vi "Get Element Description Variant.vi"(8 "error in (no error)":errorcluster, 9 "Prepend Array Size":bool=TRUE, 11 "Data Type":variant) -> (0 "error out (no error)":errorcluster, 2 "Total Size":u32, 3 "Encoder Data":T1)   [LabVIEW 2021, in "CIF_NI_CIPC.lvlib"]
uses:
  CIF_NI_CIPC.lvlib
  TypeDefs/Encoder Info.ctl
  TypeDefs/Errors.ctl
  <vilib>/CIF Foundation/CIF Utilities/Errors/Append Error Location.vi
  <vilib>/CIF Foundation/CIF Utilities/DataTypes/DataTypes_CIF_U.lvlib
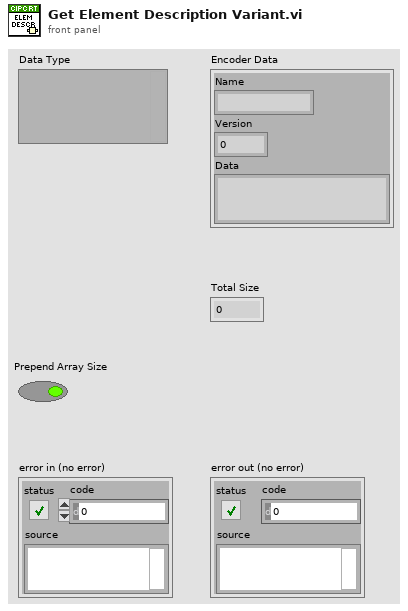
[diagram p1: front panel]
types:
  T1 = typedef "CIF_NI_CIPC.lvlib/Encoder Info.ctl" = cluster{"Name":string, "Version":i32, "Data":string}
  T2 = typedef "DataTypes_CIF_U.lvlib/Cluster Info.ctl" = cluster{"Name":string[], "Indices":i32[], "Type":T3, "Flat Data Size":u32, "Flat Data Offset":u32, "Memory Size":u32, "Memory Padding":u32, "Memory Offset":u32, "Type Descriptor":i16[]}
  T3 = typedef "NI_Data Type.lvlib/Data Type.ctl" = enum8{"Invalid Type", "Void", "I8", "I16", "I32", "I64", "U8", "U16", "U32", "U64", "Single Float", "Double Float", "Extended Float", "Single Complex", "Double Complex", "Extended Complex", "Enum U8", "Enum U16", "Enum U32", "Enum U64", "Single Float With Unit", "Double Float With Unit", "Extended Float With Unit", "Single Complex with Unit", "Double Complex with Unit", "Extended Complex with Unit", "Boolean", "String", "Path", "Picture", "Tag", "Array", "Cluster", "Variant", "LV Variant", "Waveform", "Timestamp", "Digital Waveform", "Digital Data", "ExpressData", "Refnum", "External Data", "VI", "Poly VI", "LabVIEW Class Instance", "Fixed Point", "Set Collection", "Map Collection"}
  T4 = typedef "CIF_NI_CIPC.lvlib/Errors.ctl" = enum16{"Invalid Pack Length", "Invalid Pack Destination", "Unsupported Type", "Missing Library"}
  T5 = typedef "DataTypes_CIF_U.lvlib/Endian.ctl" = enum16{"Little Endian", "Big Endian"}
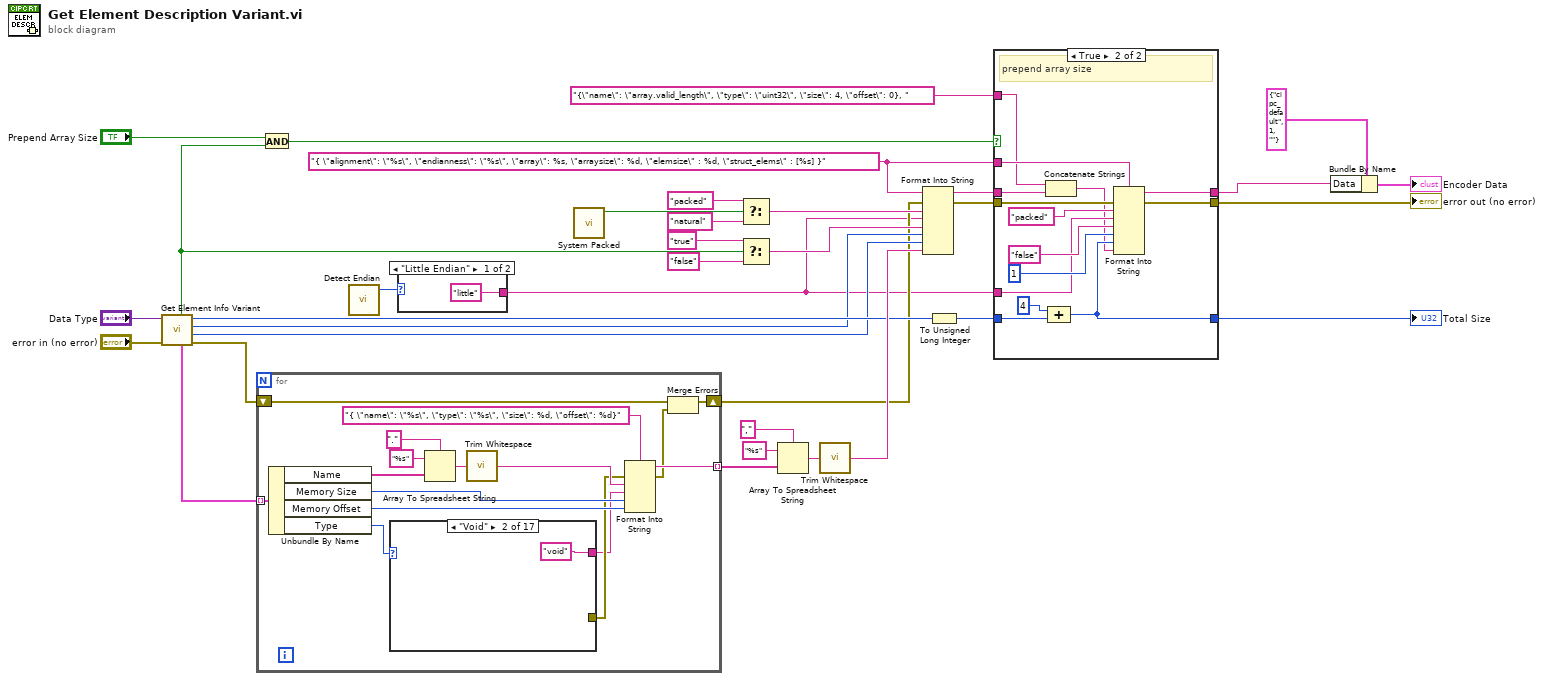
[diagram p0: block diagram]
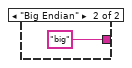
[diagram p2: hidden frame]
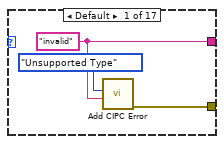
[diagram p4: hidden frame]
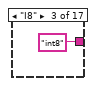
[diagram p5: hidden frame]
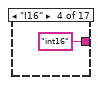
[diagram p6: hidden frame]
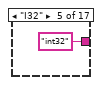
[diagram p7: hidden frame]
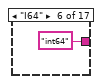
[diagram p8: hidden frame]
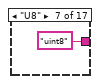
[diagram p9: hidden frame]
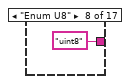
[diagram p10: hidden frame]
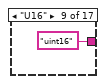
[diagram p11: hidden frame]
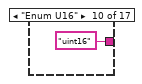
[diagram p12: hidden frame]
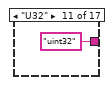
[diagram p13: hidden frame]
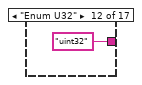
[diagram p14: hidden frame]
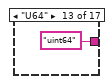
[diagram p15: hidden frame]
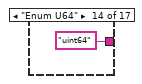
[diagram p16: hidden frame]
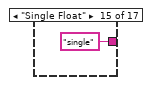
[diagram p17: hidden frame]
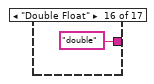
[diagram p18: hidden frame]
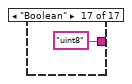
[diagram p19: hidden frame]
diagram:
  w26 = "{ \"alignment\": \"%s\", \"endianness\": \"%s\", \"array\": %s, \"arraysize\": %d, \"elemsize\" : %d, \"struct_elems\" : [%s] }" ("format string")
  n1 = call "Get Element Info Variant.vi"("error in (no error)"="error in (no error)", "Data Type"="Data Type") -> ("error out"=w9:errorcluster, "Array Element Size"=w20:i32, "Array Size"=w21:i32, "Total Size"=w22:i32, "Cluster Info"=w19:T2[], "Array"=w15:bool)  [unwired: 4 in]
  n2 = for {
    tunnel: w19 -> [w51] mode=indexing
    tunnel: [w44] -> w31 mode=indexing
    shift-right: [w42] -> w8
    shift-left: w9 -> [w40]
    n3 = Unbundle By Name(w51) -> ("Name"=w50:string[], "Memory Size"=w46:u32, "Memory Offset"=w45:u32, "Type"=w38:T3)
    n4 = case shown="\"Void\"" w38 {
      tunnel: [w52 "void" "int8" "int16" "int32" "int64" "uint8" "uint8" "uint16" "uint16" "uint32" "uint32" "uint64" "uint64" "single" "double" "uint8"] -> w36
      tunnel: [w54 _ _ _ _ _ _ _ _ _ _ _ _ _ _ _ _] -> w37
      frame Default {
        w52 = "invalid"
        n5 = call "Add CIPC Error.vi"("String to Append"=w52, "Error"=Errors."Unsupported Type") -> ("error out"=w54:errorcluster)  [unwired: 9 in]
      }
      frame "Void" {
      }
      frame "I8" {
      }
      frame "I16" {
      }
      frame "I32" {
      }
      frame "I64" {
      }
      frame "U8" {
      }
      frame "Enum U8" {
      }
      frame "U16" {
      }
      frame "Enum U16" {
      }
      frame "U32" {
      }
      frame "Enum U32" {
      }
      frame "U64" {
      }
      frame "Enum U64" {
      }
      frame "Single Float" {
      }
      frame "Double Float" {
      }
      frame "Boolean" {
      }
    }
    n6 = Array To Spreadsheet String(delimiter (Tab)=".", array=w50, 3:"%s" ("format string")) -> (spreadsheet string=w48:string)
    n7 = call <vilib>:"Trim Whitespace.vi"("string"=w48) -> ("trimmed string"=w47:string)  [unwired: 1 in]
    n8 = Format Into String(format string="{ \"name\": \"%s\", \"type\": \"%s\", \"size\": %d, \"offset\": %d}", error in=w37, w47, w36, w46, w45) -> (resulting string=w44:string, error out=w41:errorcluster)  [unwired: 1 in]
    n9 = Merge Errors(w40, w41) -> (w42:errorcluster)
  }
  n10 = And(x="Prepend Array Size", y=w15) -> (x .and. y?=w27:bool)
  n11 = call <vilib>:"Detect Endian.vi"() -> ("Endian"=w4:T5)  [unwired: 5 in]
  n12 = case shown="\"Little Endian\"" w4 {
    tunnel: ["little" "big"] -> w3
    frame "Little Endian" {
    }
    frame "Big Endian" {
    }
  }
  n13 = call <vilib>:"System Packed.vi"() -> ("packed_clusters"=w11:bool)  [unwired: 10 in, 1 out]
  n14 = Select(t="packed", s=w11, f="natural") -> (s? t:f=w12:string)
  n15 = Select(t="true", s=w15, f="false") -> (s? t:f=w16:string)
  n16 = Array To Spreadsheet String(delimiter (Tab)=",", array=w31, 3:"%s" ("format string")) -> (spreadsheet string=w32:string)
  n17 = call <vilib>:"Trim Whitespace.vi"("string"=w32) -> ("trimmed string"=w29:string)  [unwired: 1 in]
  n18 = Format Into String(format string=w26, error in=w8, w12, w3, w16, w21, w20, w29) -> (resulting string=w25:string, error out=w7:errorcluster)  [unwired: 1 in]
  n19 = To Unsigned Long Integer(number=w22) -> (unsigned 32bit integer=w5:u32)
  n20 = case shown="True" w27 {
    tunnel: w26 -> [_ w89]
    tunnel: w5 -> [w74 w85]
    tunnel: w25 -> [w75 w78]
    tunnel: [w75 w83] -> w6
    tunnel: [w73 w80] -> w24
    tunnel: [w74 w82] -> w23
    tunnel: w7 -> [w73 w81]
    tunnel: w3 -> [_ w79]
    tunnel: "{\"name\": \"array.valid_length\", \"type\": \"uint32\", \"size\": 4, \"offset\": 0}, " -> [_ w77]
    frame False {
    }
    frame True {
      # "prepend array size"
      n21 = Concatenate Strings(w77, w78) -> (w76:string)
      n22 = Compound Arithmetic op=ADD(u32 4 ("x"), w85) -> (w82:u32)
      n23 = Format Into String(format string=w89, error in=w81, "packed" ("input 1"), w79, "false" ("input 3"), 1 ("input 4"), w82, w76) -> (resulting string=w83:string, error out=w80:errorcluster)  [unwired: 1 in]
    }
  }
  "error out (no error)" <- w24
  "Total Size" <- w23
  n24 = Bundle By Name(cluster=T1 {"Name"="cipc_default", "Version"=1, "Data"=""} ("el_enc_info"), "Data"=w6) -> (→"Encoder Data":T1)
